vi "Temperature Warnings.vi"() -> ()   [LabVIEW 2018]
doc: "이 VI는 현재 온도 및 리미트 셋팅에 기반하여 기상 관측기에 출력할 문자열을 결정하는데 사용됩니다.\n\n입력: 현재 온도(DBL), 최저 온도(DBL) 및 최고 온도(DBL).\n출력: 경고 텍스트(문자열) 및 경고?(불리언)."
panel:
  in  "기상 데이터 입력":T1={"현재 온도"=0.0, "최고 온도"=0.0, "최저 온도"=0.0, "경고?"=FALSE, "경고 텍스트"="경고 없음", "단위"=enum."섭씨"}
  out "기상 데이터 출력":T1={"현재 온도"=0.0, "최고 온도"=0.0, "최저 온도"=0.0, "경고?"=FALSE, "경고 텍스트"="경고 없음", "단위"=enum."섭씨"}
  out "에러 출력":cluster{"상태":bool, "코드":i32, "소스":string}
  in  "에러 입력":cluster{"상태":bool, "코드":i32, "소스":string}
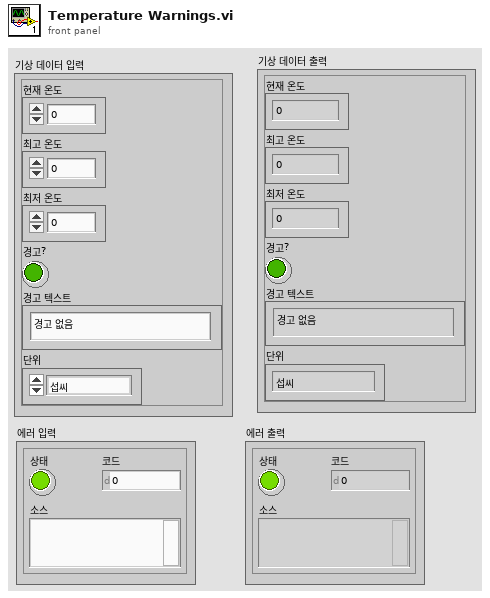
[diagram p1: front panel]
types:
  T1 = typedef "컨트롤 4.ctl" = cluster{"현재 온도":dbl, "최고 온도":dbl, "최저 온도":dbl, "경고?":bool, "경고 텍스트":string, "단위":enum16{"섭씨", "화씨", ""}}
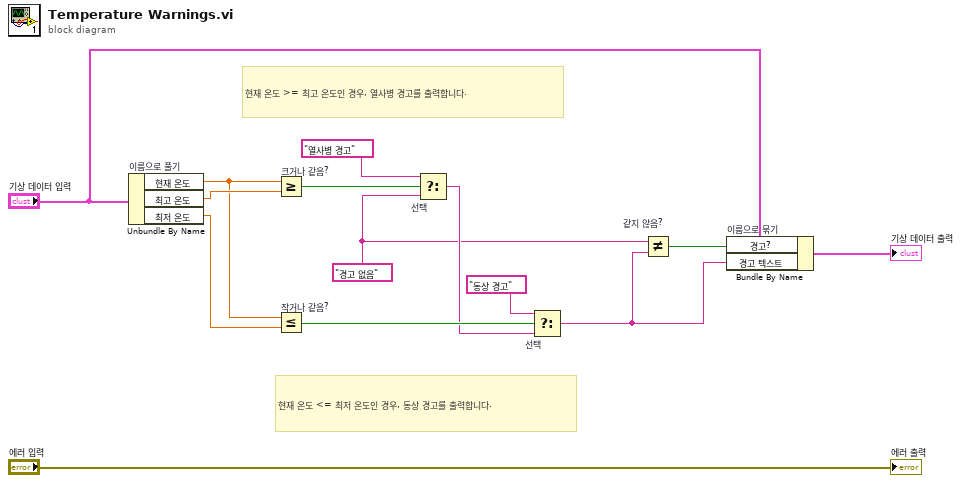
[diagram p0: block diagram]
diagram:
  w9 = "경고 없음" ("f")
  # "현재 온도 >= 최고 온도인 경우, 열사병 경고를 출력합니다."
  # "현재 온도 <= 최저 온도인 경우, 동상 경고를 출력합니다."
  n1 = Unbundle By Name "이름으로 풀기"("기상 데이터 입력") -> ("현재 온도"=w5:dbl, "최고 온도"=w7:dbl, "최저 온도"=w6:dbl)
  n2 = Greater Or Equal? "크거나 같음?"(x=w5, y=w7) -> (x >= y?=w14:bool)
  n3 = Less Or Equal? "작거나 같음?"(x=w5, y=w6) -> (x <= y?=w11:bool)
  n4 = Select "선택"(t="열사병 경고", s=w14, f=w9) -> (s? t:f=w10:string)
  n5 = Select "선택"(t="동상 경고", s=w11, f=w10) -> (s? t:f=w3:string)
  n6 = Not Equal? "같지 않음?"(x=w9, y=w3) -> (x != y?=w4:bool)
  n7 = Bundle By Name "이름으로 묶기"(cluster="기상 데이터 입력", "경고?"=w4, "경고 텍스트"=w3) -> (→"기상 데이터 출력":T1)
  "에러 출력" <- "에러 입력"
